vi "Launch Async.vi"(7 "VolatusAPI":refnum<class "VolatusAPI.lvclass">, 8 "error in (no error)":errorcluster, 10 "Value":bool, 11 "HtmlButtonControl in":refnum<class "HttpButtonControl.lvclass">) -> (0 "error out":errorcluster, 3 "HtmlButtonControl out":refnum<class "HttpButtonControl.lvclass">)   [LabVIEW 2020, in "VolatusGUIElements.lvlib" / "HttpButtonControl.lvclass"]
uses:
  HttpButtonControl.lvclass
  HttpButtonControl.lvclass/HttpButtonControl.ctl
  Do HTML Async.vi
  Volatus/VolatusAPI/VolatusAPI.lvclass
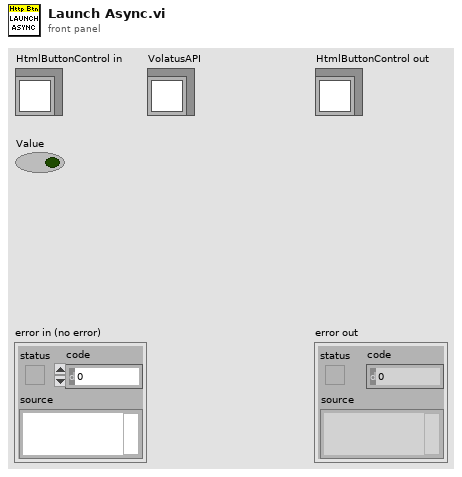
[diagram p1: front panel]
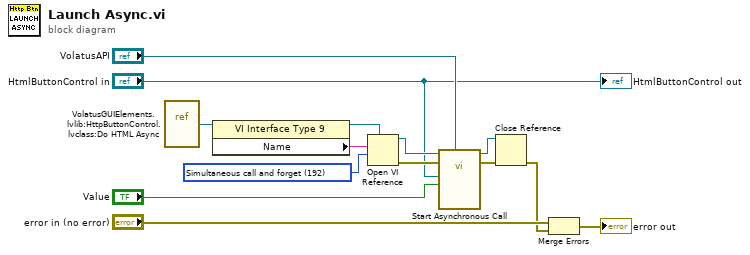
[diagram p0: block diagram]
diagram:
  w8 = 192 items=["Record modifications"=1, "Open templates for editing"=2, "Prompt user to save"=4, "Prepare for reentrant run"=8, "Prompt to find missing subVIs"=16, "Hide loading dialog box"=32, "Enable simultaneous calls"=64, "Prepare to call and forget"=128, "Simultaneous call and forget"=192, "Prepare to call and collect"=256, "Simultaneous call and collect"=320]
  n1 = vi-ref "VolatusGUIElements.lvlib:HttpButtonControl.lvclass:Do HTML Async.vi"() -> (w6:refnum<vi>)
  n2 = property class="VI Interface Type 9"(reference=w6) -> (reference out=w9:refnum<vi>, "Name"=w7:string)  [unwired: 1 in, 1 out]
  n3 = Open VI Reference(type specifier VI Refnum (for type only)=w9, vi path=w7, options=w8) -> (vi reference=w11:refnum<vi>, error out=w10:errorcluster)  [unwired: 3 in]
  n4 = call-by-ref "Start Asynchronous Call"(reference=w11, error in=w10, "VolatusAPI"="VolatusAPI", "Value"="Value", "HtmlButtonControl in"="HtmlButtonControl in") -> (reference out=w13:refnum<vi>, error out=w12:errorcluster)  [unwired: 9 in]
  n5 = Close Reference(reference=w13, error in (no error)=w12) -> (error out=w2:errorcluster)
  n6 = Merge Errors("error in (no error)", w2) -> (→"error out":errorcluster)
  "HtmlButtonControl out" <- "HtmlButtonControl in"
